vi "Can Teardown Create.vi"(8 "Error in":errorcluster, 10 "Actor in":refnum<class "Actor.lvclass">) -> (1 "Teardown Create":bool, 2 "Actor out":refnum<class "Actor.lvclass">)   [LabVIEW 2020, in "jettl.lvlib" / "Actor.lvlib"]
uses:
  Actor.lvlib
  Actor/Actor.lvclass
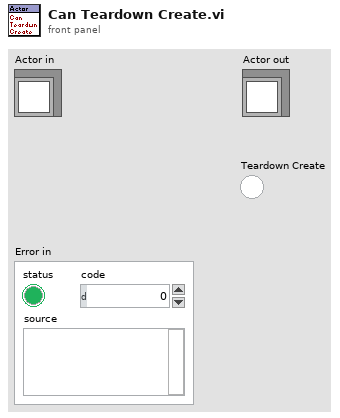
[diagram p1: front panel]
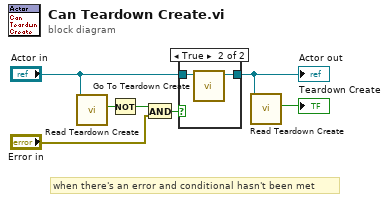
[diagram p0: block diagram]
diagram:
  # "when there's an error and conditional hasn't been met"
  n1 = call-dynamic "Read Teardown Create.vi"("Actor in"="Actor in") -> ("Teardown Create"=w4:bool)  [unwired: 10 in]
  n2 = Not(x=w4) -> (.not. x?=w7:bool)
  n3 = And(x=w7, y="Error in") -> (x .and. y?=w6:bool)
  n4 = case shown="True" w6 {
    tunnel: [w8 w9] -> w2
    tunnel: "Actor in" -> [w8 w10]
    frame False {
    }
    frame True {
      n5 = call-dynamic "Go To Teardown Create.vi"("Actor in"=w10) -> ("Actor out"=w9:refnum<class "Actor.lvclass">)  [unwired: 10 in]
    }
  }
  "Actor out" <- w2
  n6 = call-dynamic "Read Teardown Create.vi"("Actor in"=w2) -> ("Teardown Create"=→"Teardown Create":bool)  [unwired: 10 in]
